vi "CalculateDiscount.vi"(8 "Error In":errorcluster, 9 "CurrentDiscount":ext, 10 "Customer":refnum<class "Customer.lvclass">, 11 "reference in":refnum<class "ReferredCustomerRule.lvclass">) -> (0 "Error Out":errorcluster, 2 "Return(EXT)":ext, 3 "reference out":refnum<class "ReferredCustomerRule.lvclass">)   [LabVIEW 2020, in "ReferredCustomerRule.lvclass"]
uses:
  ReferredCustomerRule.lvclass
  Customer_class/Customer.lvclass
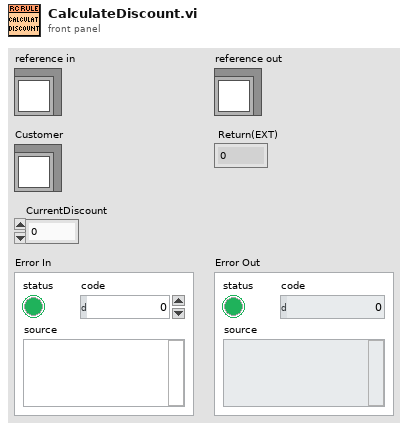
[diagram p1: front panel]
types:
  T1 = typedef "ReferredCustomerRule.lvclass/ObjectAttributes.ctl" = cluster{"PriorityLowestExecutesFirst":i32}
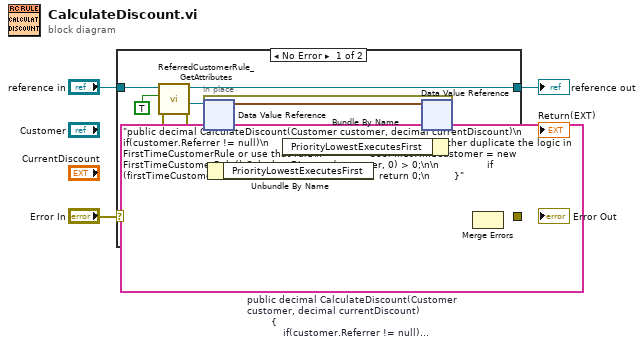
[diagram p0: block diagram]
diagram:
  (unwired) "public decimal CalculateDiscount(Customer customer, decimal currentDiscount)\n        {\n            if(customer.Referrer != null)\n            {\n                // here we can either duplicate the logic in FirstTimeCustomerRule or use that rule\n                bool firstTimeCustomer = new FirstTimeCustomerRule().CalculateDiscount(customer, 0) > 0;\n\n                if (firstTimeCustomer) return .30m;\n            }\n            return 0;\n        }"  # public decimal CalculateDiscount(Customer customer, decimal currentDiscount)         {             if(customer.Referrer != null)             {                 // here we can either duplicate the logic in FirstTimeCustomerRule or use that rule                 bool firstTimeCustomer = new FirstTimeCustomerRule().CalculateDiscount(customer, 0) > 0;                  if (firstTimeCustomer) return .30m;             }             return 0;         }
  n1 = case shown="No Error" "Error In" {
    selector: "Error In" -> [w11 w16]
    tunnel: [w8 w16] -> w3
    tunnel: [w9 w15] -> w1
    tunnel: "reference in" -> [w12 w15]
    frame No Error {
      n2 = call "ReferredCustomerRule_GetAttributes.vi"("error in (no error)"=w11, "OnlyGetDvrReference(False)"=TRUE, "reference in"=w12) -> ("error out"=w6:errorcluster, "DataRef"=w7:refnum<data-value>, "reference out"=w9:refnum<class "ReferredCustomerRule.lvclass">)  [unwired: 5 in, 1 out]
      n3 = in-place {
        n4 = in-place-dvr #1(w7) -> (w13:T1)  [unwired: 1 out]
        n5 = Unbundle By Name(w13) -> ()  [unwired: 1 out]
        n6 = Bundle By Name(cluster=w13) -> (w14:T1)  [unwired: 1 in]
        n7 = in-place-dvr #1(w14) -> (w10:errorcluster)  [unwired: 1 out]
      }
      n8 = Merge Errors(w6, w10) -> (w8:errorcluster)
    }
    frame Error {
    }
  }
  "Error Out" <- w3
  "reference out" <- w1
